vi "Instantiate LV Dev.vi"   [LabVIEW 2016, in "LV Doc.lvclass"]
uses:
  LV Doc.lvclass
  Child Classes/LV DEV/LV DEV.lvclass
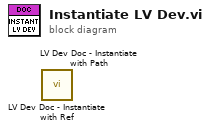
[diagram p0: block diagram]
diagram:
  n1 = call "LV Dev Doc - Instantiate with Ref.vi"() -> ()  [unwired: 14 in, 2 out]
  n2 = call "LV Dev Doc - Instantiate with Path.vi"() -> ()  [unwired: 14 in, 2 out]
